vi "Clear sound buffer.vi"(8 "error in (no error)":errorcluster, 10 "array":T1[](array[typedef]) format="%.0x", 11 "task ID":T1 format="%.0x") -> (0 "error out":errorcluster)   [LabVIEW 2019]
uses:
  <vilib>/sound2/lvsound2.llb/Sound Output Task ID.ctl
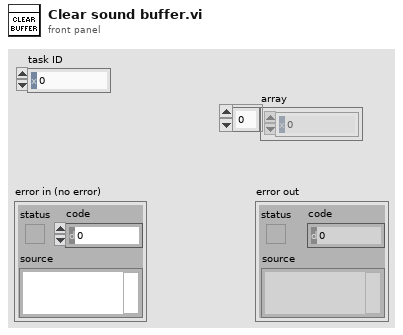
[diagram p1: front panel]
types:
  T1 = typedef "Sound Output Task ID.ctl" = u32
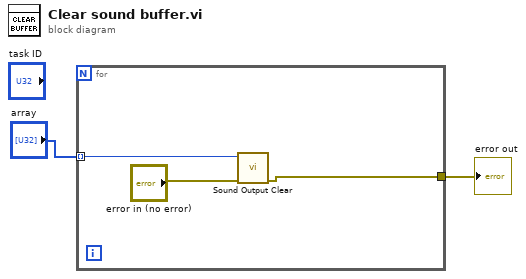
[diagram p0: block diagram]
diagram:
  n1 = for {
    tunnel: "array" -> [w4] mode=indexing
    tunnel: [w3] -> w1
    n2 = call <vilib>:"Sound Output Clear.vi"("error in (no error)"="error in (no error)", "task ID"=w4) -> ("error out"=w3:errorcluster)  [unwired: 9 in]
  }
  "error out" <- w1
